vi "Seconds Breakdown.vi"(11 "全部时间（秒）":dbl) -> (0 "消息":string, 1 "秒":dbl, 2 "分钟":dbl, 3 "小时":dbl, 5 "警告":bool)   [LabVIEW 2012]
panel:
  # "将秒数转换成小时、分钟和秒的独立显示。\n如果时间超过1小时，通过LED和消息向用户报警。"
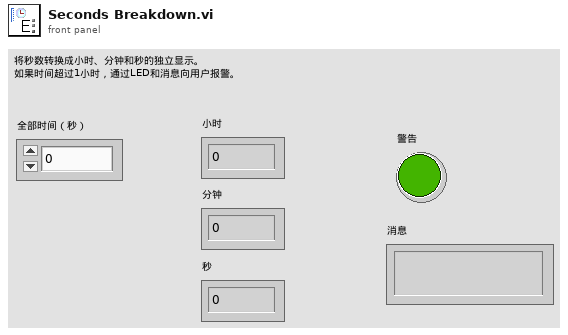
[diagram p1: front panel]
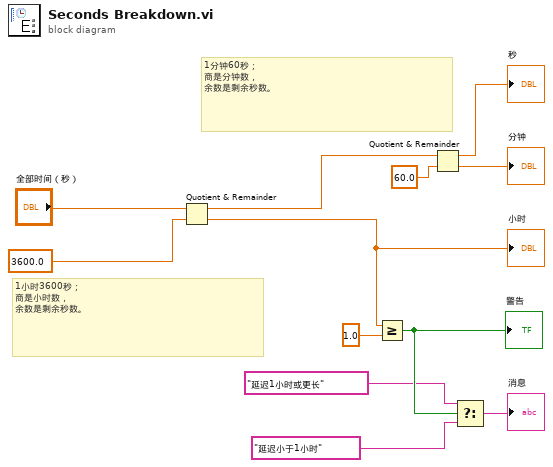
[diagram p0: block diagram]
diagram:
  # "1分钟60秒；\n商是分钟数，\n余数是剩余秒数。"
  # "1小时3600秒；\n商是小时数，\n余数是剩余秒数。"
  n1 = Quotient & Remainder ("商与余数")(x="全部时间（秒）", y=3600.0) -> (x-y*floor(x/y)=w11:dbl, floor(x/y)=w6:dbl)
  "小时" <- w6
  n2 = Greater Or Equal? ("大于等于？")(x=w6, y=1.0) -> (x >= y?=w4:bool)
  "警告" <- w4
  n3 = Quotient & Remainder ("商与余数")(x=w11, y=60.0) -> (x-y*floor(x/y)=→"秒":dbl, floor(x/y)=→"分钟":dbl)
  n4 = Select ("选择")(t="延迟1小时或更长", s=w4, f="延迟小于1小时") -> (s? t:f=→"消息":string)
